vi "trace_math_spectra_absorbance2.vi"(0 "reference in":refnum<class "OSA.lvclass">, 1 "spectrum sample trace idx":u32, 2 "spectrum bgrnd trace idx":u32, 3 "spectrum abso trace idx":u32, 5 "error in (no error)":errorcluster) -> (13 "global absorbance trace idx":u32, 14 "reference out":refnum<class "OSA.lvclass">, 19 "error out":errorcluster)   [LabVIEW 2010, in "OSA.lvclass"]
doc: "Calculates a absorbance spectrum from a sample and a background spectrum The 'sample' and 'background' spectra must both be of the type 'SPEC_EMISSION' \n\nParameters\n\nsample: the spectrum of the sample to calculate the absorbance of.\n\nbackground: the spectrum to use as background spectrum \n\nabsorbance: will on successful return be filled with the calculated absorbance."
uses:
  OSA.lvclass
  typeDef/acq_dataType.ctl
  FTSLib.dll
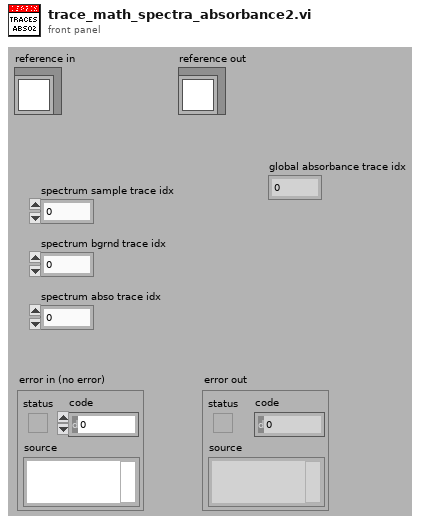
[diagram p1: front panel]
types:
  T1 = typedef "OSA.lvclass/acq_dataType.ctl" = enum16{"none", "interferogram", "spectrum"}
  T2 = typedef "OSA.lvclass/ObjectAttributes.ctl" = cluster{"Stop":bool, "dataType":T1, "spectrometerIdx":u16, "buffer size interferogram":i32, "interferogram":cluster{"new":bool, "plot_x_ min":sgl, "plot_x_max":sgl, "plot_y_min":sgl, "plot_y_max":sgl, "Graph Intrfrgrm":T3, "timeStamp":u32, "signal (%)":dbl, "traces":cluster{"idx":u32, "broadBand":bool, "monoChromatic":bool, "peakToPeakSignal":dbl, "peakToPeakPos":dbl}[], "traces idx last":i32}, "spectrum":cluster{"new":bool, "plot_x_min":sgl, "plot_x_max":sgl, "plot_unit_x":T4, "plot_unit_y":T5, "plot_y_min":sgl, "plot_y_max":sgl, "Graph Spectrum":T3, "timeStamp":u32, "X_VAL_OPTIONS":enum16{"MIN_MAX", "ARRAY"}, "traces":cluster{"idx":u32}[], "traces idx last":i32}, "Thorlabs_OSA_64.lvclass:queue_action.ctlqueue ref":refnum<queue>, "action":T6, "plot zoom step":dbl, "buffer semaphore":T7, "acq stopped":bool, "dataType active":T1, "temperature (degr C)":sgl, "pressure (hPa)":sgl, "rel humidity (%)":sgl, "settings":cluster{"resolution":u16, "sensitivity":u16, "Average":bool, "average nr":u32, "apodisation":T8, "acq delay (ms)":u32, "airMesure":T9, "wmtr on":bool, "intfgrm_smooth_width":u16, "intfgrm_smooth_nrOfPasses":u16, "intfgrm_smooth":T10, "phaseCorrection":T11, "zeroFill":u8, "spectr_smooth":T10, "spectr_smooth_width":u16, "spectr_smooth_nrOfPasses":u16, "resolution (/cm)":sgl, "REF wavelength, (nm)":dbl, "gain_idx":u16, "gainAuto":bool, "gain_relative":dbl, "PD sensitivity mode":T12, "PD senseMode implemented":bool, "SensorTemperature implemented":bool, "SensorPressure implemented":bool, "SensorHumidity implemented":bool}, "peaks position":sgl[], "peaks width":sgl[], "peaks height":sgl[], "peaks max nr":u32, "peaks latest nr":i32, "peaks new":bool, "power":dbl, "power new":bool, "path":string, "wavelength (WNr)":dbl, "wavelength new":bool, "buffer size spectrum":i32, "status":string, "VI reference":refnum<vi>, "funcPointer":u64, "libraryPointer":u64, "singleAcquisition":bool, "coherenceLength (cm)":dbl, "coherenceLength new":bool, "spectrometer model":string, "spectrometer serial nr":string, "peaks thld left":sgl[], "peaks thld right":sgl[], "coherenceLength error (cm)":dbl, "ADC bits":u16, "peaks position centroid":sgl[], "peaks height centroid":sgl[], "OSA series":T13, "channel index spectrum":u16, "spectrometer rangeLow, (/cm)":dbl, "spectrometer rangeHigh, (/cm)":dbl, "channel index interferogram":u16}
  T3 = typedef "OSA.lvclass/graph_intensity.ctl" = refnum<vi>
  T4 = typedef "OSA.lvclass/spectrum_x_unit.ctl" = enum16{"wavenr/cm", "THz", "eV", "nm_air", "nm_vac"}
  T5 = typedef "OSA.lvclass/y_unit.ctl" = enum16{"ADC counts", "dBm pwr absolute", "dBm pwr density", "mW pwr absolute", "mW pwr density"}
  T6 = typedef "OSA.lvclass/queue_action.ctl" = enum16{"none", "stop", "GUI_plotInterferogram", "GUI_plotSpectrum", "GUI_plotInterferogramRescale", "GUI_plotSpectrumRescale", "GUI_plotInterferogramReset", "GUI_plotSpectrumReset", "GUI_plotInterferogramAutoScaleY", "GUI_plotSpectrumAutoScaleY", "GUI_plotInterferogramZoomOut", "GUI_plotSpectrumZoomOut", "GUI_plotInterferogramPane", "GUI_plotSpectrumPane", "GUI_plotInterferogramZoomMouse", "GUI_plotSpectrumZoomMouse", "ENVIRONMENT temperature", "ENVIRONMENT pressure", "MODE_resolution set", "MODE_resolution get", "MODE_sensitivity set", "MODE_sensitivity get", "MODE_PDTemperature set", "MODE_PDTemperature get", "REBOOT/RESET firmware", "ACQASYNC_acquireSingleSpectrum", "ACQASYNC_continuous start", "ACQASYNC_continuous stop\n", "ACQASYNC_get last interferogram", "ACQASYNC_get last spectrum", "ACQASYNC_get last waveNr", "ACQOPT_interferogram smoothing set", "ACQOPT_interferogram smoothing get", "ACQOPT_spectrum smoothing set", "ACQOPT_spectrum smoothing get", "ACQOPT_apodisation type set", "ACQOPT_apodisation type get", "ACQOPT_phase correction type set", "ACQOPT_phase correction type get", "ACQOPT_acqIntervall_set", "ACQOPT_acqIntervall_get", "ACQOPT_average spectrum set", "ACQOPT_average spectrum get", "ACQOPT_rolling average set", "ACQOPT_rolling average get", "ACQOPT_zero fill factor set", "ACQOPT_zero fill factor get", "ACQOPT_cycle counting set", "ACQOPT_cycle counting get", "ACQOPT_air measure option set", "ACQOPT_air measure option get", "ACQOPT_gainLevel auto get", "ACQOPT_gainLevel auto set", "ACQOPT_gainLevel get", "ACQOPT_gainLevel set", "ACQOPT_getAll", "INSTRUMENT_PROPERTY_range_WaveNr_min", "INSTRUMENT_PROPERTY_range_WaveNr_max", "INSTRUMENT_PROPERTY_reference_wavelength_cm^-1", "INSTRUMENT_PROPERTY_samplesPerRefPeriod", "INSTRUMENT_PROPERTY_resolution_waveNrPercm", "INSTRUMENT_PROPERTY_availableGainLevels", "INSTRUMENT_PROPERTY_status", "CONVERT", "ANALYSE_POWER", "ANALYSE_PEAKS", "ANALYSE_WAVELENGTH", "ANALYSE_SPECTRUM", "ANALYSE_INTERFEROGRAM", "ANALYSE_COHERENCE_LENGTH", "MATH", "MATH_power", "MATH_peaks", "FILE", "miscellaneous"}
  T7 = typedef "Semaphore RefNum" = refnum<k1>
  T8 = typedef "OSA.lvclass/apodisation.ctl" = enum16{"NONE", "NORTON_BEER_WEAK", "NORTON_BEER_MEDIUM", "NORTON_BEER_STRONG", "TRIANGULAR", "COSINE", "HANN", "HAMMING", "BLACKMANHARRIS3", "BLACKMANHARRIS4", "GAUSSIAN"}
  T9 = typedef "OSA.lvclass/airMeasure.ctl" = enum16{"TEMPERATURE", "PRESSURE"}
  T10 = typedef "OSA20X_misc.lvlib/interferogram_smoothing.ctl" = enum16{"NONE", "BINOMIAL", "SAVITSKY_GOLAY", "FOURIER", "MOVING_AVERAGE", "GAUSSIAN"}
  T11 = typedef "OSA.lvclass/phaseCorrection.ctl" = enum16{"NONE", "MERTZ", "FORMAN", "MERTZ_FILE", "FORMAN_FILE", "FUTURE COMP."}
  T12 = typedef "OSA20X_misc.lvlib/PDTemperatureMode.ctl" = enum16{"cool: better sensitivity/noise floor", "warm: extended wl range"}
  T13 = typedef "OSA.lvclass/OSA_series.ctl" = enum16{"OSA200", "OSA300", "UNKNOWN"}
  T14 = cluster{"idx":u32, "broadBand":bool, "monoChromatic":bool, "peakToPeakSignal":dbl, "peakToPeakPos":dbl}[]
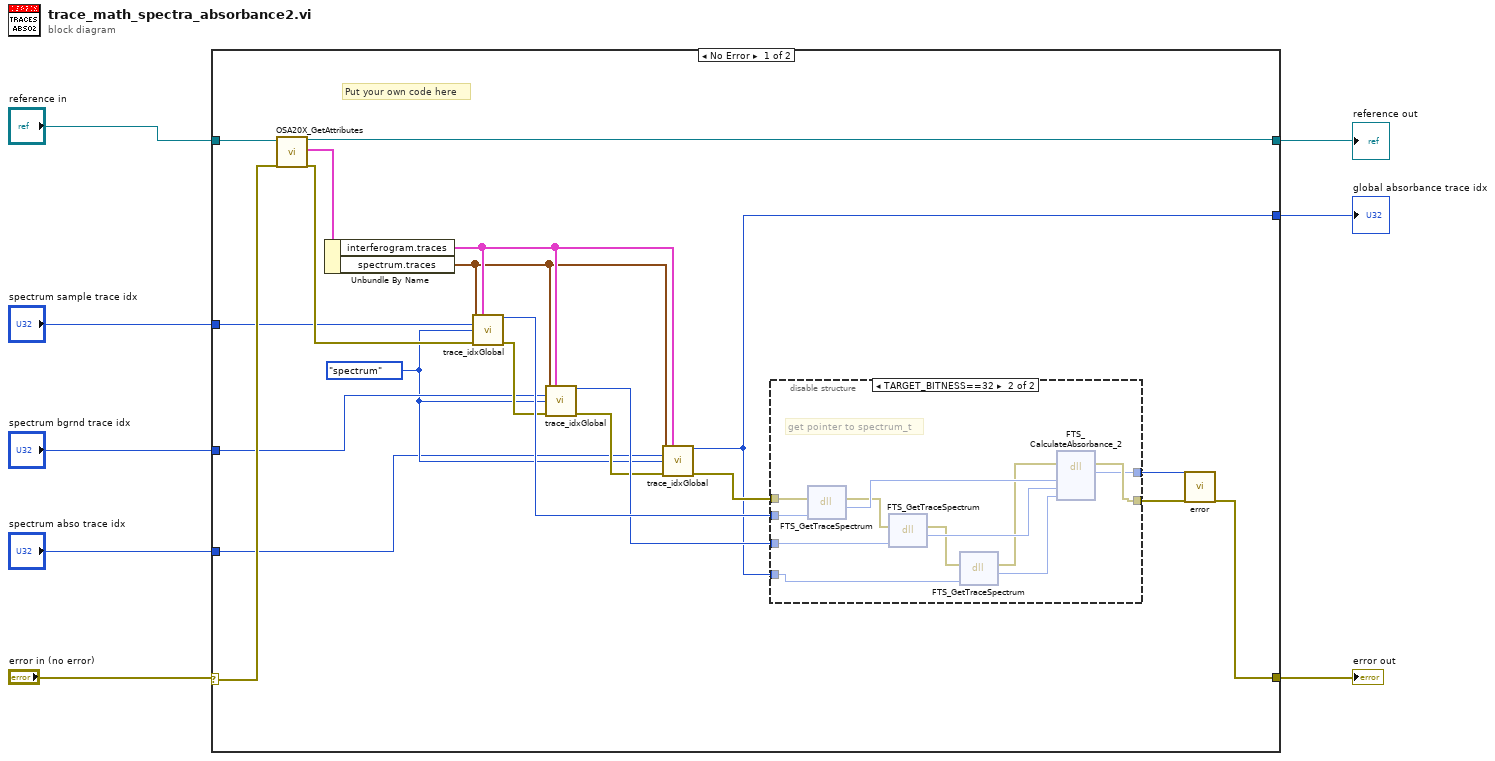
[diagram p0: block diagram]
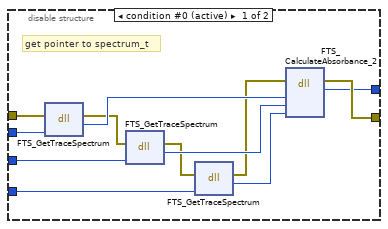
[diagram p2: hidden frame]
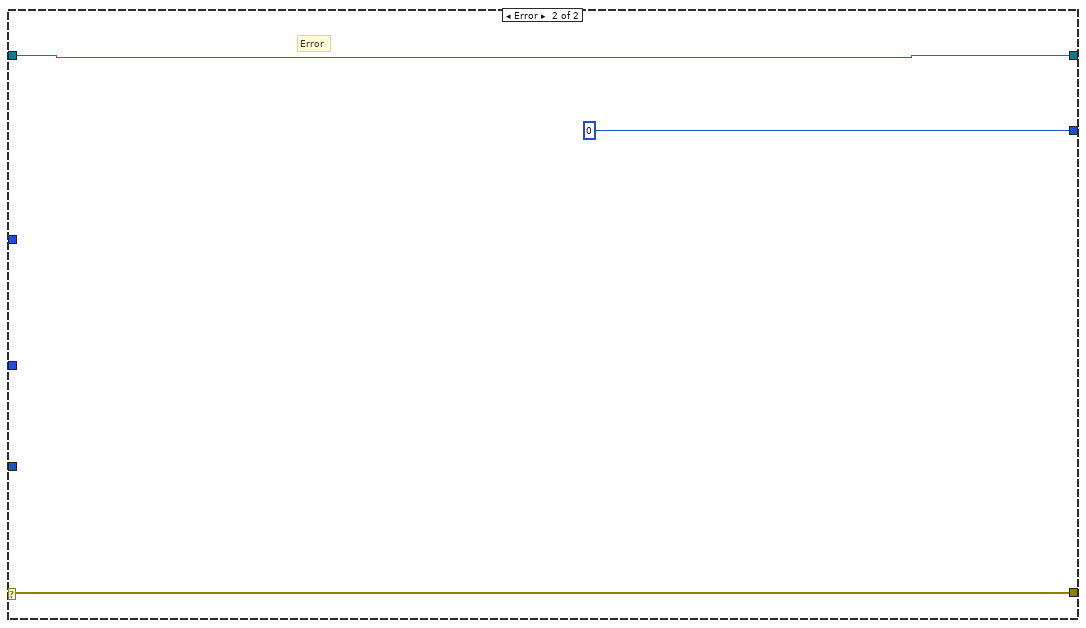
[diagram p3: hidden frame]
diagram:
  n1 = case shown="No Error" "error in (no error)" {
    selector: "error in (no error)" -> [w24 w55]
    tunnel: [w28 w55] -> w8
    tunnel: "reference in" -> [w26 w54]
    tunnel: [w25 w54] -> w3
    tunnel: "spectrum sample trace idx" -> [w22 _]
    tunnel: [w9 u32 0 ("global trace idx")] -> w4
    tunnel: "spectrum bgrnd trace idx" -> [w17 _]
    tunnel: "spectrum abso trace idx" -> [w10 _]
    frame No Error {
      w11 = acq_dataType."spectrum" ("dataType")
      # "Put your own code here"
      n2 = call "OSA20X_GetAttributes.vi"("reference in"=w26, "error in (no error)"=w24) -> ("reference out"=w25:refnum<class "OSA.lvclass">, "Data"=w27:T2, "error out"=w23:errorcluster)  [unwired: 14 in, 1 out]
      n3 = Unbundle By Name(w27) -> ("interferogram.traces"=w15:T14, "spectrum.traces"=w14:cluster{"idx":u32}[])
      n4 = call "trace_idxGlobal.vi"("traces_spectrum"=w14, "traces_interferogram"=w15, "trace idx"=w22, "dataType"=w11, "error in (no error)"=w23) -> ("global trace idx"=w19:u32, "error out"=w18:errorcluster)  [unwired: 9 in]
      n5 = call "trace_idxGlobal.vi"("traces_spectrum"=w14, "traces_interferogram"=w15, "trace idx"=w17, "dataType"=w11, "error in (no error)"=w18) -> ("global trace idx"=w16:u32, "error out"=w13:errorcluster)  [unwired: 9 in]
      n6 = call "trace_idxGlobal.vi"("traces_spectrum"=w14, "traces_interferogram"=w15, "trace idx"=w10, "dataType"=w11, "error in (no error)"=w13) -> ("global trace idx"=w9:u32, "error out"=w12:errorcluster)  [unwired: 9 in]
      n7 = disable-structure shown="TARGET_BITNESS==32" {
        disable-tunnel: w19 -> [w40 w46]
        disable-tunnel: w12 -> [w38 w47]
        disable-tunnel: [w37 w49] -> w21
        disable-tunnel: [w36 w48] -> w20
        disable-tunnel: w16 -> [w34 w45]
        disable-tunnel: w9 -> [w30 w41]
        frame condition #0 (active) {
          # "get pointer to spectrum_t"
          n8 = dll-call lib="FTSLib.dll" fn="FTS_GetTraceSpectrum"(error in=w38, "traceIdx"=w40) -> (error out=w35:errorcluster, "spectrum_t_pointer"=w39:u64)  [unwired: 3 in, 1 out]
          n9 = dll-call lib="FTSLib.dll" fn="FTS_GetTraceSpectrum"(error in=w35, "traceIdx"=w34) -> (error out=w32:errorcluster, "spectrum_t_pointer"=w33:u64)  [unwired: 3 in, 1 out]
          n10 = dll-call lib="FTSLib.dll" fn="FTS_GetTraceSpectrum"(error in=w32, "traceIdx"=w30) -> (error out=w31:errorcluster, "spectrum_t_pointer"=w29:u64)  [unwired: 3 in, 1 out]
          n11 = dll-call lib="FTSLib.dll" fn="FTS_CalculateAbsorbance_2"(error in=w31, "spectrum_t_pointer"=w39, "spectrum_t_pointer"=w33, "spectrum_t_pointer"=w29) -> (error out=w37:errorcluster, "returnVal"=w36:i32)  [unwired: 5 in, 1 out]
        }
        frame condition #1 {
          # "get pointer to spectrum_t"
          n12 = dll-call lib="FTSLib.dll" fn="FTS_GetTraceSpectrum"(error in=w47, "traceIdx"=w46) -> (error out=w51:errorcluster, "spectrum_t_pointer"=w52:u32)  [unwired: 3 in, 1 out]
          n13 = dll-call lib="FTSLib.dll" fn="FTS_GetTraceSpectrum"(error in=w51, "traceIdx"=w45) -> (error out=w44:errorcluster, "spectrum_t_pointer"=w50:u32)  [unwired: 3 in, 1 out]
          n14 = dll-call lib="FTSLib.dll" fn="FTS_GetTraceSpectrum"(error in=w44, "traceIdx"=w41) -> (error out=w43:errorcluster, "spectrum_t_pointer"=w42:u32)  [unwired: 3 in, 1 out]
          n15 = dll-call lib="FTSLib.dll" fn="FTS_CalculateAbsorbance_2"(error in=w43, "spectrum_t_pointer"=w52, "spectrum_t_pointer"=w50, "spectrum_t_pointer"=w42) -> (error out=w49:errorcluster, "returnVal"=w48:i32)  [unwired: 5 in, 1 out]
        }
      }
      n16 = call "error.vi"("result code"=w20, "error in (no error)"=w21) -> ("error out"=w28:errorcluster)  [unwired: 15 in, 2 out]
    }
    frame Error {
      # "Error"
    }
  }
  "error out" <- w8
  "reference out" <- w3
  "global absorbance trace idx" <- w4
